vi "routes_n_m.vi"(8 "error in (no error)":errorcluster, 10 "m = number of nodes (horizontal)":u32, 11 "n = number of nodes (vertical)":u32) -> (0 "error out":errorcluster, 3 "r(n,m)= number of routes":u32)   [LabVIEW 2021, in "Project Euler.lvlib"]
uses:
  Project Euler.lvlib
panel:
  # "Development\ncontrols/indicators useful for development and testing, but which are not outputs of the VI"
  # "Input\nInputs to the VI"
  # "Output\nOutputs of the VI"
  # "Description\n\nBlank VI with error handling case. \n\nSummarize the use of this VI in this space."
  # "r(15,15) = 40,116,600\nr(16,16) = 155,117,520\nr(17,17) = 601,080,390"
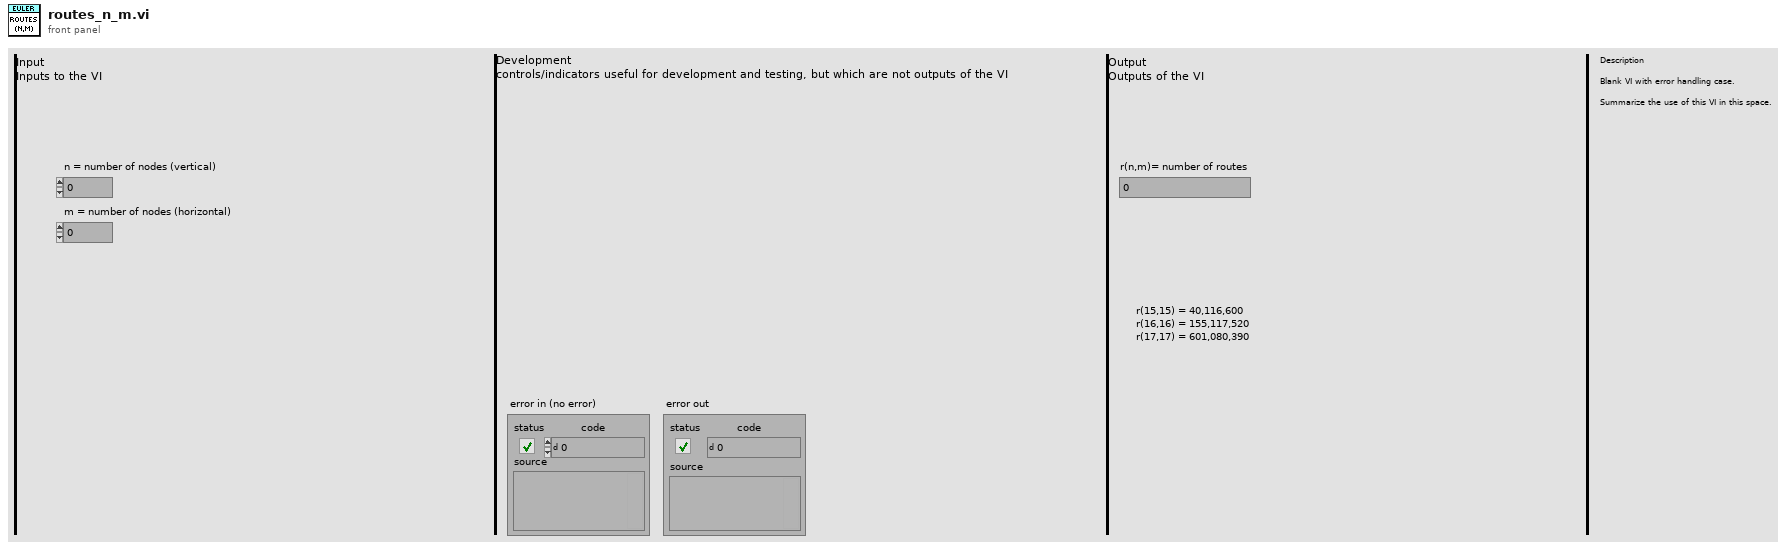
[diagram p1: front panel]
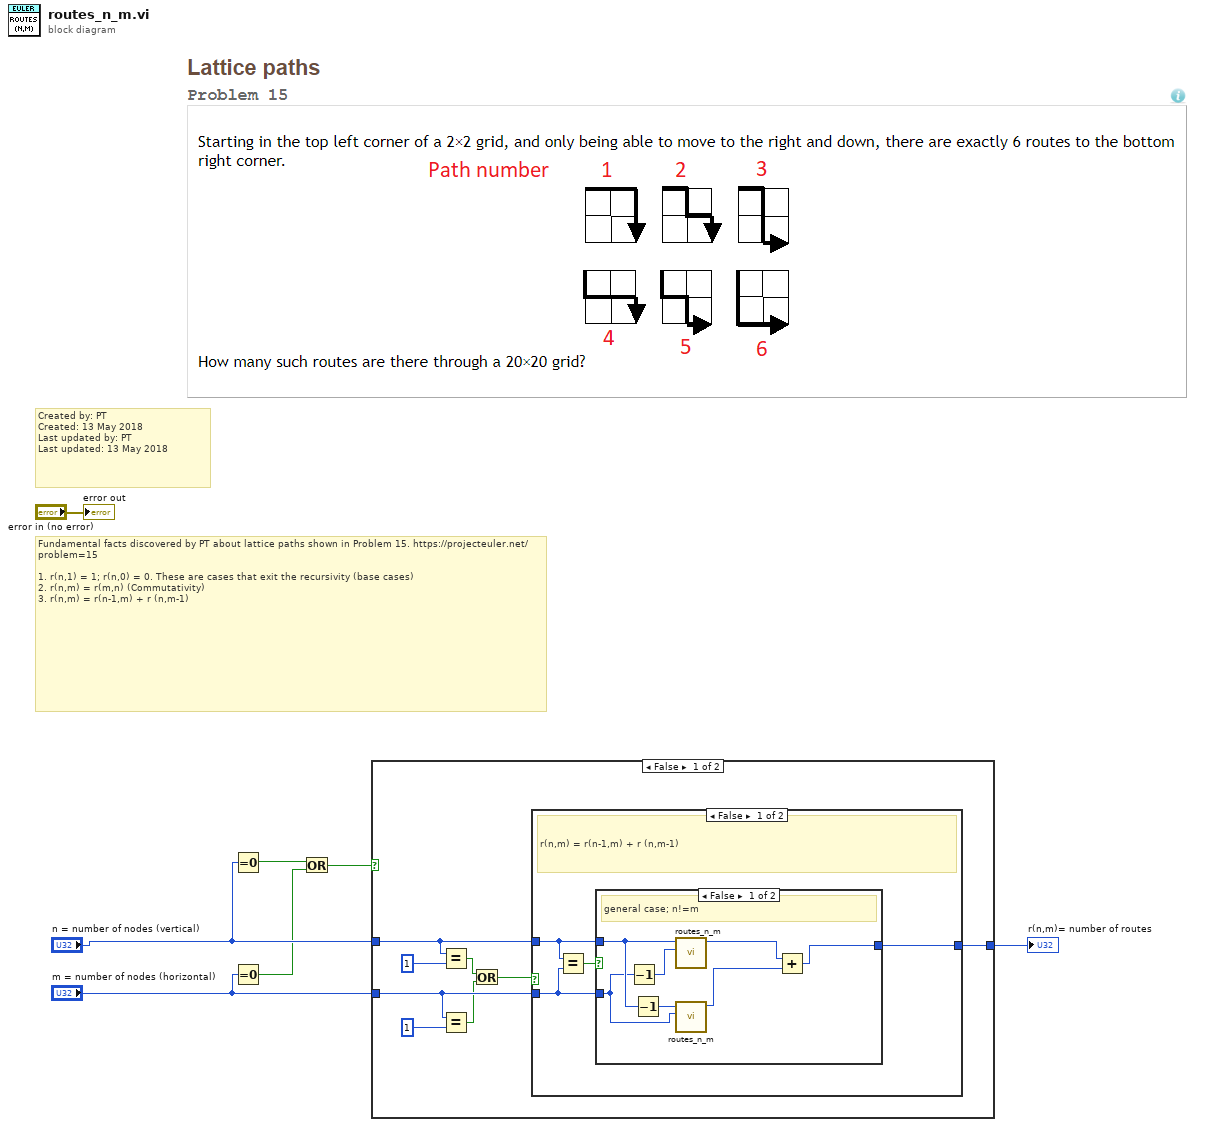
[diagram p0: block diagram]
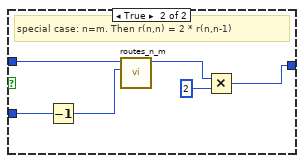
[diagram p2: hidden frame]
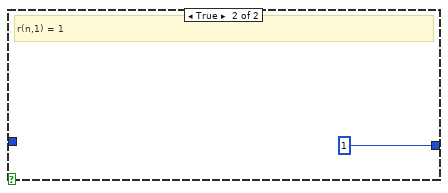
[diagram p3: hidden frame]
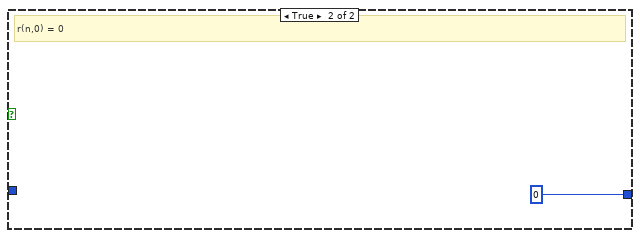
[diagram p4: hidden frame]
diagram:
  # "Fundamental facts discovered by PT about lattice paths shown in Problem 15. https://projecteuler.net/problem=15\n\n1. r(n,1) = 1; r(n,0) = 0. These are cases that exit the recursivity (base cases)\n2. r(n,m) = r(m,n) (Commutativity)\n3. r(n,m) = r(n-1,m) + r (n,m-1)"
  # "Created by: PT\nCreated: 13 May 2018\nLast updated by: PT\nLast updated: 13 May 2018"
  n1 = Equal To 0?(x="n = number of nodes (vertical)") -> (x = 0?=w3:bool)
  n2 = Equal To 0?(x="m = number of nodes (horizontal)") -> (x = 0?=w2:bool)
  n3 = Or(x=w3, y=w2) -> (x .or. y?=w1:bool)
  n4 = case shown="False" w1 {
    tunnel: [w15 u32 0 ("r(n,m)= number of routes")] -> w6
    tunnel: "n = number of nodes (vertical)" -> [w14 _]
    tunnel: "m = number of nodes (horizontal)" -> [w10 _]
    frame False {
      n5 = Equal?(x=w14, y=u32 1) -> (x = y?=w12:bool)
      n6 = Equal?(x=w10, y=u32 1) -> (x = y?=w9:bool)
      n7 = Or(x=w12, y=w9) -> (x .or. y?=w8:bool)
      n8 = case shown="False" w8 {
        tunnel: w14 -> [w18 _]
        tunnel: w10 -> [w17 _]
        tunnel: [w19 u32 1 ("r(n,m)= number of routes")] -> w15
        frame False {
          # "r(n,m) = r(n-1,m) + r (n,m-1)"
          n9 = Equal?(x=w18, y=w17) -> (x = y?=w16:bool)
          n10 = case shown="False" w16 {
            tunnel: w18 -> [w23 w32]
            tunnel: w17 -> [w21 w31]
            tunnel: [w20 w27] -> w19
            frame False {
              # "general case; n!=m"
              n11 = Decrement(x=w21) -> (x-1=w26:u32)
              n12 = Decrement(x=w23) -> (x-1=w22:u32)
              n13 = call "routes_n_m.vi"("m = number of nodes (horizontal)"=w26, "n = number of nodes (vertical)"=w23) -> ("r(n,m)= number of routes"=w25:u32)  [unwired: 8 in, 1 out]
              n14 = call "routes_n_m.vi"("m = number of nodes (horizontal)"=w21, "n = number of nodes (vertical)"=w22) -> ("r(n,m)= number of routes"=w24:u32)  [unwired: 8 in, 1 out]
              n15 = Add(x=w25, y=w24) -> (x+y=w20:u32)
            }
            frame True {
              # "special case: n=m. Then r(n,n) = 2 * r(n,n-1)"
              n16 = Decrement(x=w31) -> (x-1=w30:u32)
              n17 = call "routes_n_m.vi"("m = number of nodes (horizontal)"=w30, "n = number of nodes (vertical)"=w32) -> ("r(n,m)= number of routes"=w29:u32)  [unwired: 8 in, 1 out]
              n18 = Multiply(x=w29, y=u32 2) -> (x*y=w27:u32)
            }
          }
        }
        frame True {
          # "r(n,1) = 1"
        }
      }
    }
    frame True {
      # "r(n,0) = 0"
    }
  }
  "r(n,m)= number of routes" <- w6
  "error out" <- "error in (no error)"
